vi "Colin_Fun.vi"(10 "Old Files":T2[](array[typedef])) -> ()   [LabVIEW 2022 SP3]
uses:
  Curtin1_Label.ctl
  <vilib>/Utility/miscctls.llb/LVRangeTypeDef.ctl
  <vilib>/Native 3D Graph/xcontrol/3DPC_SurfacePlot.xctl
panel:
  in  "Plots":enum32{"2D", "3D"}(tab)
  out "Nyquist Plot":cluster{dbl[], dbl[]}(graph)
  out "3D Nyquist":refnum<class "Base Datatype.lvclass">[](xcontrol)
  out "NewRange":T1
  out "Energy":cluster{"x0":dbl, "df":dbl, dbl[]}[](graph)
  in  "Data Set":u16(ring) items=["JacksonStrad H.AvC", "JacksonStrad H.AvC", "JacksonStrad V.AvC", "JacksonStrad V.AvC", "Roberto Jardon - BBar 1 rad H.AvC", "Roberto Jardon - BBar 1 rad V.AvC", "Roberto Jardon - BBar 2 rad H.AvC", "Roberto Jardon - BBar 2 rad V.AvC", "Roberto Jardon - Transverse Bar 3 H.AvC", "Roberto Jardon - Transverse Bar 3 V.AvC"]
  # "Welcome to George's Plots\n\nThese allow one to see the real and imaginary parts of the signal.  Select the particular run you want to visualize.  Make sure you have selected the complex averages and not the real averages (as they do not have a complex part)"
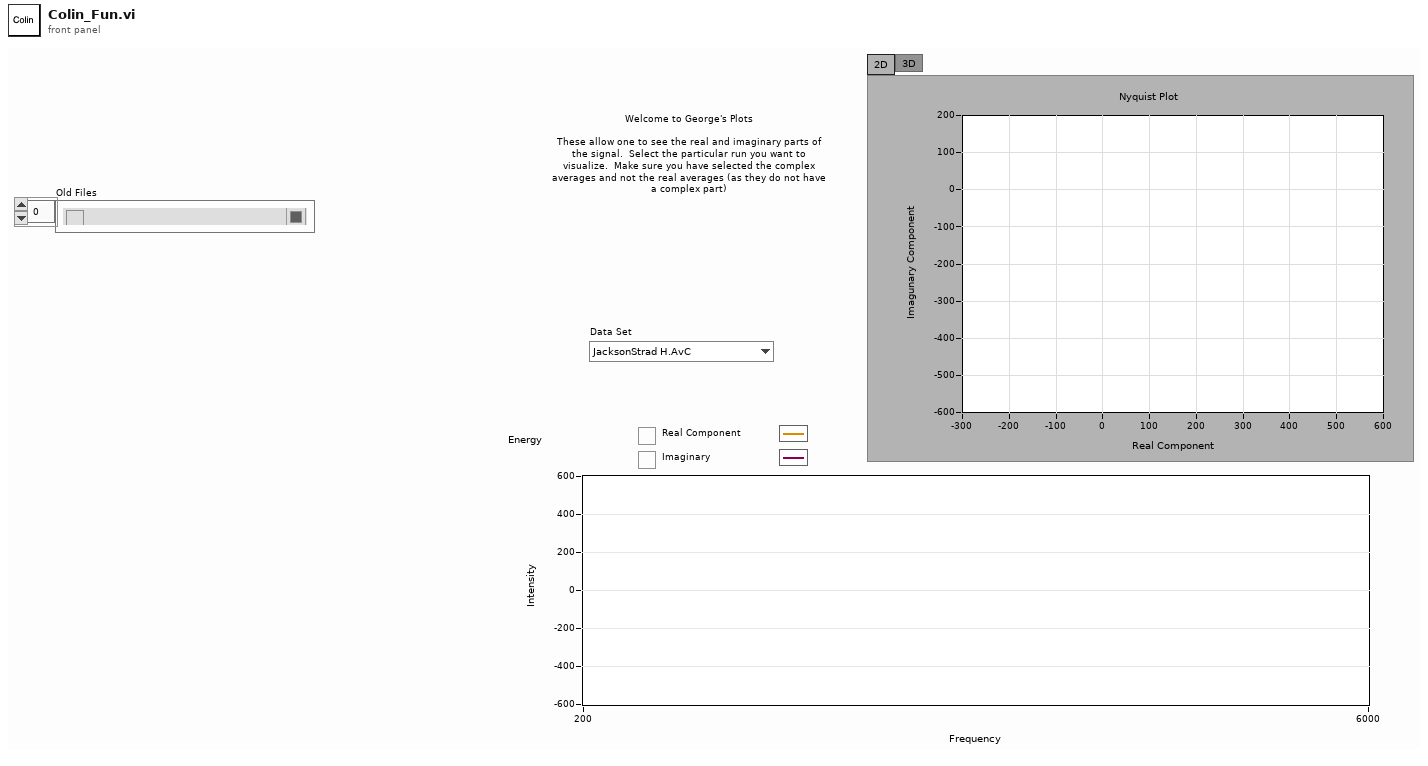
[diagram p1: front panel]
types:
  T1 = typedef "LVRangeTypeDef.ctl" = cluster{"Minimum":dbl, "Maximum":dbl, "Increment":dbl, "Minor Increment":dbl, "Start":dbl}
  T2 = typedef "Curtin1_Label.ctl" = cluster{"Show?":bool, "Name":string, "Color":u32, "Path":path, "Show Notes":bool}
  T3 = cluster{"Start freq":dbl, "Hz resolution":dbl, cdb[]}
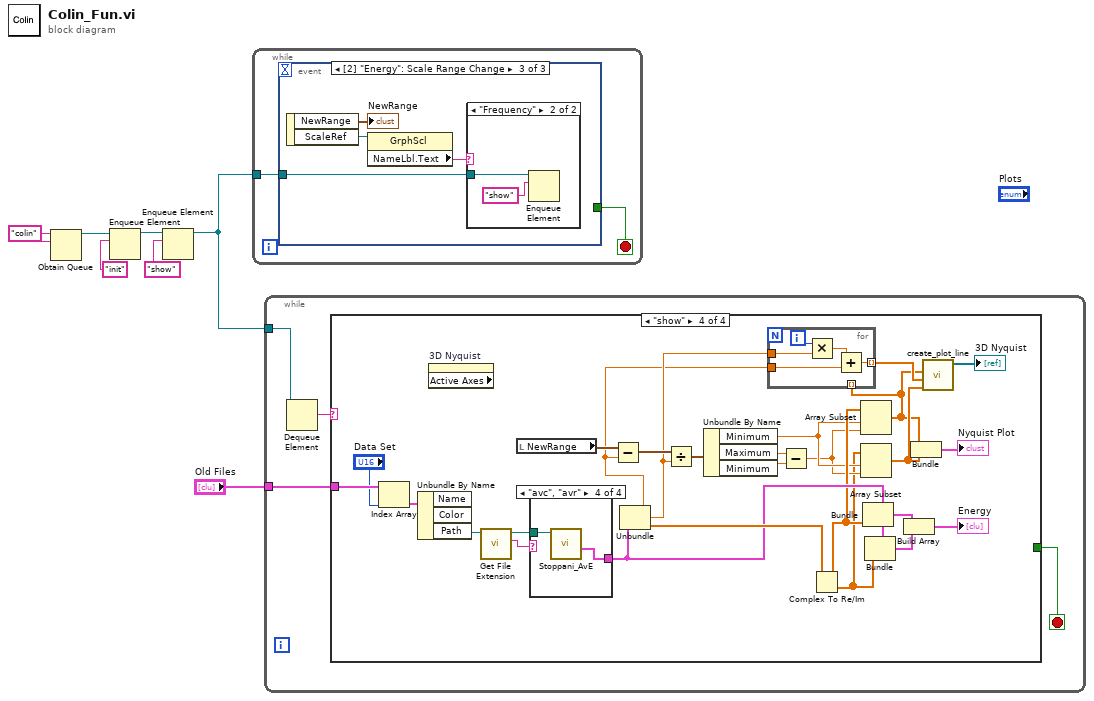
[diagram p0: block diagram]
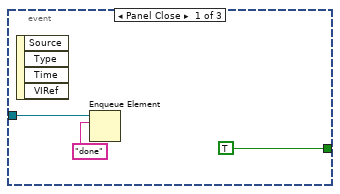
[diagram p2: hidden frame]
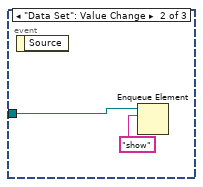
[diagram p3: hidden frame]
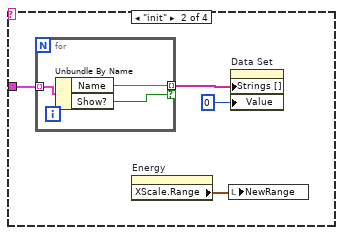
[diagram p6: hidden frame]
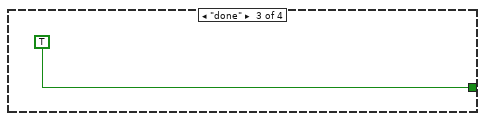
[diagram p7: hidden frame]
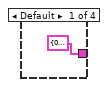
[diagram p8: hidden frame]
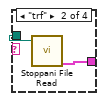
[diagram p9: hidden frame]
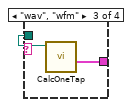
[diagram p10: hidden frame]
diagram:
  w7 = "colin" ("name (unnamed)")
  n1 = Obtain Queue(name (unnamed)=w7, element data type=w7) -> (queue out=w2:refnum<queue>)  [unwired: 3 in, 2 out]
  n2 = Enqueue Element(queue=w2, element="init") -> (queue out=w1:refnum<queue>)  [unwired: 2 in, 2 out]
  n3 = Enqueue Element(queue=w1, element="show") -> (queue out=w5:refnum<queue>)  [unwired: 2 in, 2 out]
  n4 = while {
    tunnel: w5 -> [w8]
    stop <- w9 stop-if-true
    n5 = event shown="[2] \"Energy\": Scale Range Change" {
      selector: _ -> [_ _ _]
      dyn-events: _ -> [_ _ _]
      timeout: _ -> [_ _ _]
      tunnel: [TRUE _ _] -> w9
      tunnel: w8 -> [w10 w13 w18]
      event Panel Close {
        n6 = event-data() -> ()  [unwired: 1 in, 4 out]
        n7 = Enqueue Element(queue=w10, element="done") -> ()  [unwired: 2 in, 3 out]
      }
      event "Data Set": Value Change {
        n8 = event-data() -> ()  [unwired: 1 in, 1 out]
        n9 = Enqueue Element(queue=w13, element="show") -> ()  [unwired: 2 in, 3 out]
      }
      event "Energy": Scale Range Change {
        n10 = event-data() -> ("NewRange"=→"NewRange":T1, "ScaleRef"=w16:refnum<vi>)  [unwired: 1 in]
        n11 = property class="GrphScl"(reference=w16) -> ("NameLbl.Text"=w15:string)  [unwired: 1 in, 2 out]
        n12 = case shown="\"Frequency\"" w15 {
          tunnel: w18 -> [_ w19]
          frame "False", Default {
          }
          frame "Frequency" {
            n13 = Enqueue Element(queue=w19, element="show") -> ()  [unwired: 2 in, 3 out]
          }
        }
      }
    }
  }
  n14 = while {
    tunnel: w5 -> [w24]
    tunnel: "Old Files" -> [w21]
    stop <- w22 stop-if-true
    n15 = Dequeue Element(queue=w24) -> (element=w23:string)  [unwired: 2 in, 3 out]
    n16 = case shown="\"show\"" w23 {
      tunnel: [_ _ TRUE _] -> w22
      tunnel: w21 -> [_ w28 _ w58]
      frame Default {
      }
      frame "init" {
        n17 = for {
          tunnel: w28 -> [w31] mode=indexing
          tunnel: [w30] -> w27 mode=indexing if=w29
          n18 = Unbundle By Name(w31) -> ("Name"=w30:string, "Show?"=w29:bool)
        }
        n19 = property on="Energy" class="WFGraph (strict)"() -> ("XScale.Range"=w25:T1)  [unwired: 2 in, 2 out]
        n20 = local write "NewRange"(w25) -> ()
        n21 = property on="Data Set" class="Ring (strict)"("Strings []"=w27, "Value"=0) -> ()  [unwired: 2 in, 2 out]
      }
      frame "done" {
      }
      frame "show" {
        n22 = Index Array(array=w58, index="Data Set") -> (element=w59:T2)
        n23 = Unbundle By Name(w59) -> ("Path"=w56:path)  [unwired: 2 out]
        n24 = property on="3D Nyquist" class="LabVIEW 3D Graph (strict)" props=["Active Axes"]() -> ()  [unwired: 2 in, 3 out]
        n25 = call <vilib>:"Get File Extension.vi"("file"=w56) -> ("lowercase file extension"=w54:string, "dup file"=w55:path)  [unwired: 6 in, 3 out]
        n26 = local read "NewRange"() -> (w47:T1)
        n27 = case shown="\"avc\", \"avr\"" w54 {
          tunnel: [T3 {"Start freq"=0.0, "Hz resolution"=0.0, []} ("Waveform Graph") w66 w68 w71] -> w52
          tunnel: w55 -> [_ w67 w69 w70]
          frame Default {
          }
          frame "trf" {
            n28 = call "Stoppani File Read.vi"("String in"=w67) -> ("Complex FRF"=w66:cluster{"t0":dbl, "dt":dbl, "Y":cdb[]})  [unwired: 2 in, 3 out]
          }
          frame "wav", "wfm" {
            n29 = call "CalcOneTap.vi"("wavform file"=w69) -> ("Complex FRF"=w68:cluster{dbl, "df":dbl, cdb[]})  [unwired: 7 in, 3 out]
          }
          frame "avc", "avr" {
            n30 = call "Stoppani_AvE.vi"("file (use dialog)"=w70) -> ("Complex FRF"=w71:cluster{"t0":dbl, "df":dbl, "Y":cdb[]})  [unwired: 7 in, 3 out]
          }
        }
        n31 = Unbundle(w52) -> ("t0"=w37:dbl, "df"=w38:dbl, "Y"=w53:cdb[])
        n32 = Subtract(x=w47, y=w37) -> (x-y=w46:T1)
        n33 = Divide(x=w46, y=w38) -> (x/y=w45:T1)
        n34 = Unbundle By Name(w45) -> ("Minimum"=w42:dbl, "Maximum"=w44:dbl, "Minimum"=w33:dbl)
        n35 = Subtract(x=w44, y=w33) -> (x-y=w41:dbl)
        n36 = Complex To Re/Im(x + iy=w53) -> (x=w43:dbl[], y=w40:dbl[])
        n37 = Array Subset(array=w43, index=w42, length=w41) -> (w34:dbl[])
        n38 = for {
          tunnel: w34 -> [_] mode=indexing
          tunnel: w38 -> [w63]
          tunnel: w37 -> [w61]
          tunnel: [w60] -> w35 mode=indexing
          i -> [w64]
          n39 = Multiply(x=w64, y=w63) -> (x*y=w62:dbl)
          n40 = Add(x=w62, y=w61) -> (x+y=w60:dbl)
        }
        n41 = Array Subset(array=w40, index=w42, length=w41) -> (w36:dbl[])
        n42 = Bundle(cluster=w52, "Y"=w43) -> (w50:cluster{"t0":dbl, "df":dbl, "Y":cdb[]})  [unwired: 2 in]
        n43 = Bundle(cluster=w52, "Y"=w40) -> (w51:cluster{"t0":dbl, "df":dbl, "Y":cdb[]})  [unwired: 2 in]
        n44 = Build Array(w50, w51) -> (→"Energy":cluster{"t0":dbl, "df":dbl, "Y":cdb[]}[])
        n45 = Bundle(w34, w36) -> (→"Nyquist Plot":cluster{dbl[], dbl[]})  [unwired: 1 in]
        n46 = call <vilib>:"create_plot_line.vi"("z vector"=w36, "y vector"=w35, "x vector"=w34) -> ("plots out"=→"3D Nyquist":refnum<class "Base Datatype.lvclass">[])  [unwired: 2 in, 6 out]
      }
    }
  }
